vi "Get RPM Tast Name.vi"(8 "error in (no error)":errorcluster, 11 "Config Data":T1={"Diagnostic_Modes"={"Selected_Mode"=""}, "Basic_Health"={"Task_Name"="", "Sample_Rate_Hz"=0.0, "Samples_Per_Channel"=0, "RPM_PPR "=0.0}, "Complex_Machinery"={"Task_Name"="", "Sample_Rate_Hz"=0.0, "Samples_Per_Channel"=0, "RPM_PPR "=0.0}, "Multi_Point"={"Task_Name"="", "Sample_Rate_Hz"=0.0, "Samples_Per_Channel"=0, "RPM_PPR "=0.0}, "System_Settings"={"Simulation_Mode "="", "Options"=enum."Healthy"}, "Relay"={"Task_Name"="Local_Trip_Relay_Task"}, "RPM"={"Task_Name"="", "Max_Expected_RPM"=0.0, "Min_Expected_RPM"=0.0, "Terminal_Name"=""}}) -> (0 "error out":errorcluster, 3 "RPM Task Name":string)   [LabVIEW 2026, in "Acquisition.lvlib"]
uses:
  Controls/Vibration_Monitor_Config.ctl
  Controls/Vibration_Profile.ctl
  Controls/System_Settings.ctl
  Controls/Options.ctl
  Controls/Relay_Profile.ctl
  Controls/RPM_Profile.ctl
  Acquisition.lvlib
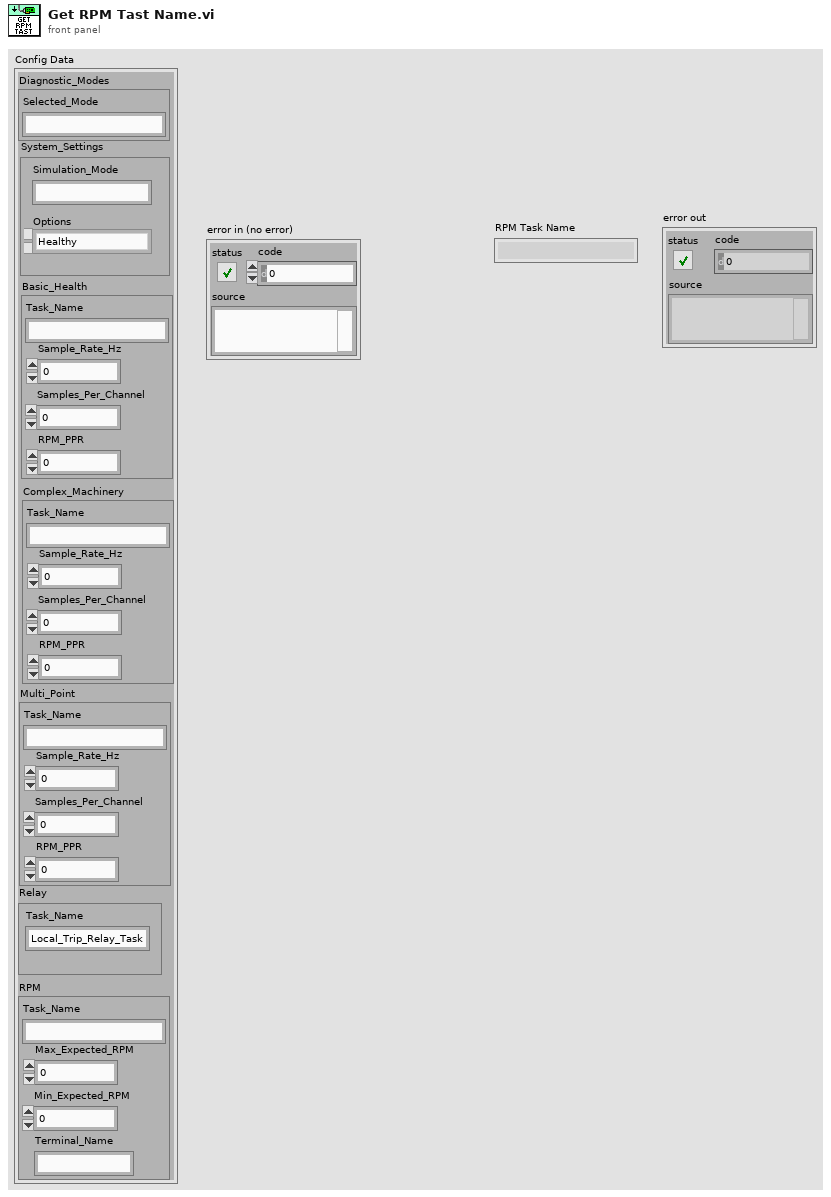
[diagram p1: front panel]
types:
  T1 = typedef "Vibration_Monitor_Config.ctl" = cluster{"Diagnostic_Modes":cluster{"Selected_Mode":string}, "Basic_Health":T2, "Complex_Machinery":T2, "Multi_Point":T2, "System_Settings":T3, "Relay":T5, "RPM":T6}
  T2 = typedef "Vibration_Profile.ctl" = cluster{"Task_Name":string, "Sample_Rate_Hz":dbl, "Samples_Per_Channel":i32, "RPM_PPR ":dbl}
  T3 = typedef "System_Settings.ctl" = cluster{"Simulation_Mode ":string, "Options":T4}
  T4 = typedef "Options.ctl" = enum16{"Healthy", "Unbalance_Alert", "Bearing_Fault_Critical", "Sweep_Test"}
  T5 = typedef "Relay_Profile.ctl" = cluster{"Task_Name":string}
  T6 = typedef "RPM_Profile.ctl" = cluster{"Task_Name":string, "Max_Expected_RPM":dbl, "Min_Expected_RPM":dbl, "Terminal_Name":string}
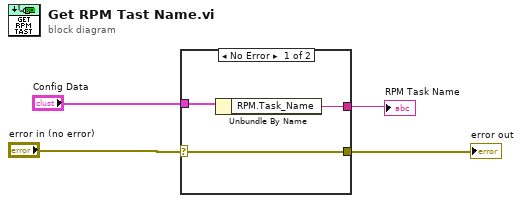
[diagram p0: block diagram]
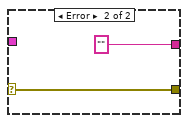
[diagram p2: hidden frame]
diagram:
  n1 = case shown="No Error" "error in (no error)" {
    selector: "error in (no error)" -> [w7 w8]
    tunnel: [w7 w8] -> w3
    tunnel: "Config Data" -> [w6 _]
    tunnel: [w5 "" ("Task_Name")] -> w1
    frame No Error {
      n2 = Unbundle By Name(w6) -> ("RPM.Task_Name"=w5:string)
    }
    frame Error {
    }
  }
  "error out" <- w3
  "RPM Task Name" <- w1
